vi "SetMeasureId.vi"(8 "error in":errorcluster, 10 "MeasureId":string, 11 "Measure in":refnum<class "Measure.lvclass">) -> (0 "error out":errorcluster, 3 "Measure out":refnum<class "Measure.lvclass">)   [LabVIEW 2021, in "ProligentXMLGenerator.lvlib" / "Measure.lvclass"]
doc: "Defines the name of the unit of the measure value (Ex: kilometer). When a unit symbol is provided, the unit name becomes required.\nDefines the symbol of the unit for the measure value (ex: km). When a unit name is provided, the unit symbol becomes required.\n\nUnit Name vaule is restricted to 30 characters and Unit Symbol is restricted to 20 characters."
uses:
  Measure.lvclass
  Measure.lvclass/Measure.ctl
  Base/Attribute/Attribute.lvclass
  Base/Guid/Guid.lvclass
  C:/Projects/proligent-xml-generator-labview/src/ProligentXMLGenerator/Base/NonEmptyString/NonEmptyString.lvclass
  C:/Projects/proligent-xml-generator-labview/src/ProligentXMLGenerator/Base/String/String.lvclass
  C:/Projects/proligent-xml-generator-labview/src/ProligentXMLGenerator/Base/Attribute/Attribute.lvclass
  C:/Projects/proligent-xml-generator-labview/src/ProligentXMLGenerator/Base/Guid/Guid.lvclass
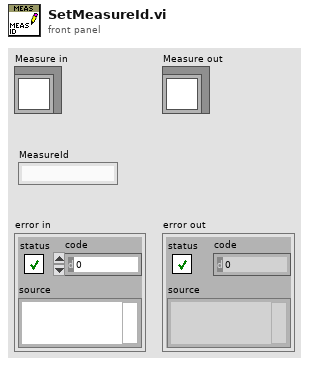
[diagram p1: front panel]
types:
  T1 = typedef "ProligentXMLGenerator.lvlib/Measure.lvclass/Data.ctl" = cluster{"Name":string, "Type":refnum<class "MeasureKind.lvclass">, "Precision":refnum<class "UnsignedByte.lvclass">, "Limit":refnum<class "MeasureLimit.lvclass">, "Characteristics":refnum<class "Characteristic.lvclass">[], "FailureReferences":refnum<class "FailureReference.lvclass">[], "CustomData":refnum<class "CustomData.lvclass">, "MeasureId":refnum<class "Guid.lvclass">, "MeasureTime":refnum<class "DateTime.lvclass">, "Comments":refnum<class "NonNullableString_TruncateAt_255.lvclass">, "Unit":refnum<class "NonEmptyString_30.lvclass">, "Symbol":refnum<class "NonEmptyString_20.lvclass">, "MeasureExecutionStatus":refnum<class "ExecutionStatus.lvclass">}
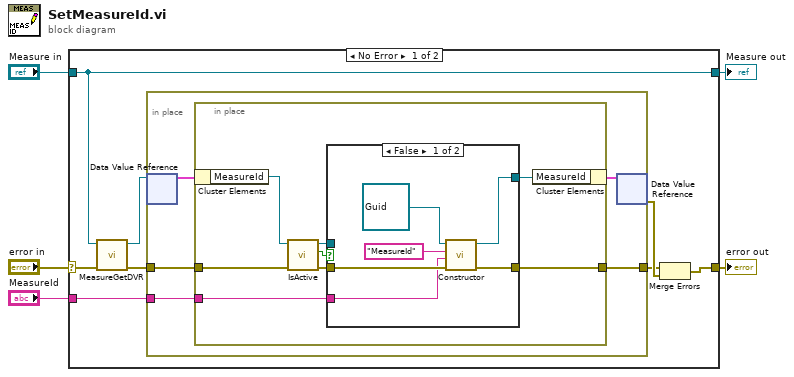
[diagram p0: block diagram]
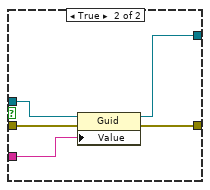
[diagram p2: hidden frame]
diagram:
  n1 = case shown="No Error" "error in" {
    selector: "error in" -> [w11 w38]
    tunnel: "Measure in" -> [w7 w39]
    tunnel: [w8 w38] -> w3
    tunnel: "MeasureId" -> [w6 _]
    tunnel: [w7 w39] -> w1
    frame No Error {
      n2 = call "MeasureGetDVR.vi"("error in"=w11, "Measure"=w7) -> ("error out"=w10:errorcluster, "DVRReference"=w12:refnum<data-value>)  [unwired: 8 in]
      n3 = in-place "In Place Element Structure" {
        in-place-border: w10 -> [w18]
        in-place-border: [w17] -> w9
        in-place-border: w6 -> [w14]
        n4 = in-place-dvr #1(w12) -> (w16:T1)  [unwired: 1 out]
        n5 = in-place "In Place Element Structure" {
          in-place-border: w18 -> [w24]
          in-place-border: [w26] -> w17
          in-place-border: w14 -> [w23]
          n6 = in-place-cluster #2(w16) -> ("MeasureId"=w25:refnum<class "Guid.lvclass">)
          n7 = call "IsActive.vi"("error in"=w24, "Attribute in"=w25) -> ("error out"=w22:errorcluster, "IsActive"=w21:bool, "Attribute in"=w20:refnum<class "Guid.lvclass">)  [unwired: 7 in]
          n8 = case shown="False" w21 {
            tunnel: w22 -> [w30 w35]
            tunnel: [w29 w34] -> w26
            tunnel: [w28 w37] -> w19
            tunnel: w20 -> [_ w36]
            tunnel: w23 -> [w27 w33]
            frame False {
              n9 = call-dynamic "Constructor.vi"("error in"=w30, "Value"=w27, "Name"="MeasureId", "String in"=refnum<class "Guid.lvclass"> refnum ("ProligentResultProcessor:NonEmptyString_30")) -> ("error out"=w29:errorcluster, "String out"=w28:refnum<class "Guid.lvclass">)  [unwired: 6 in]
            }
            frame True {
              n10 = property on="Property Node" class="Guid"(reference=w36, error in=w35, "Value"=w33) -> (reference out=w37:refnum<class "Guid.lvclass">, error out=w34:errorcluster)
            }
          }
          n11 = in-place-cluster #2("MeasureId"=w19) -> (w15:T1)
        }
        n12 = in-place-dvr #1(w15) -> (w13:errorcluster)  [unwired: 1 out]
      }
      n13 = Merge Errors(w9, w13) -> (w8:errorcluster)
    }
    frame Error {
    }
  }
  "error out" <- w3
  "Measure out" <- w1
